vi "GLOBAL -MAIN.vi"() -> ()   [LabVIEW 2015]
panel:
  out "EXIT":bool
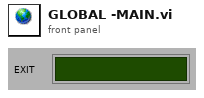
[diagram p1: front panel]
diagram:
